vi "Clear Frame Filters.vi"(8 "error in":errorcluster, 11 "IMG_SRC in":refnum<class "IMG_SRC.lvclass">) -> (0 "error out":errorcluster, 3 "IMG_SRC out":refnum<class "IMG_SRC.lvclass">)   [LabVIEW 2018, in "IMG_SRC.lvlib" / "IMG_SRC.lvclass"]
uses:
  IMG_SRC.lvclass
  IMG_SRC.lvclass/IMG_SRC.ctl
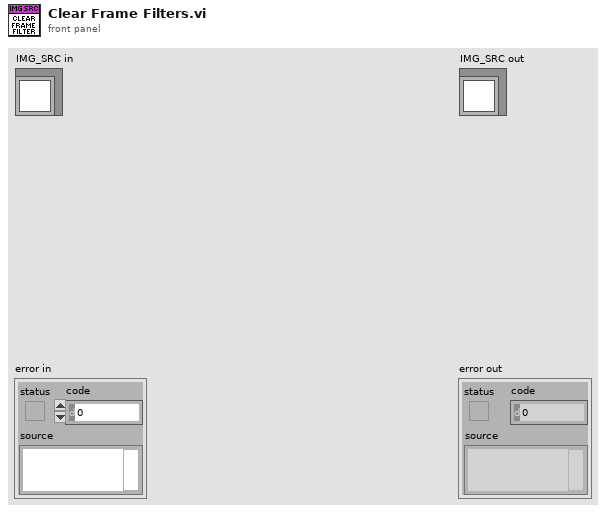
[diagram p1: front panel]
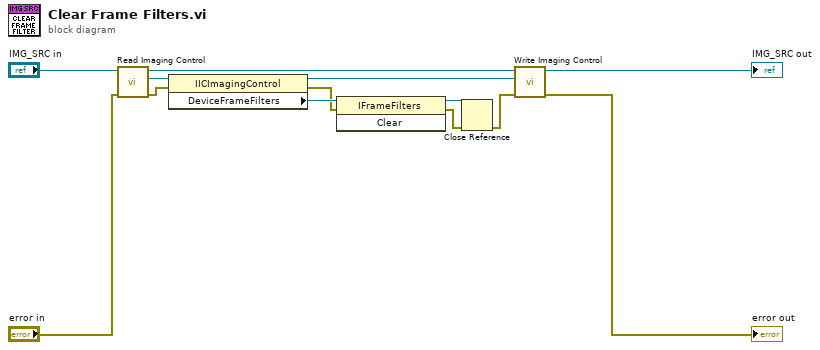
[diagram p0: block diagram]
diagram:
  n1 = call "Read Imaging Control.vi"("error in (no error)"="error in", "IMG_SRC in"="IMG_SRC in") -> ("error out"=w11:errorcluster, "Imaging Control"=w12:refnum<k7>, "IMG_SRC out"=w7:refnum<class "IMG_SRC.lvclass">)  [unwired: 7 in]
  n2 = property class="IICImagingControl"(reference=w12, error in=w11) -> (reference out=w8:refnum<k7>, error out=w9:errorcluster, "DeviceFrameFilters"=w10:refnum<k7>)
  n3 = invoke class="IFrameFilters" method="Clear"(reference=w10, error in=w9) -> (reference out=w3:refnum<k7>, error out=w2:errorcluster)  [unwired: 1 in, 1 out]
  n4 = Close Reference(reference=w3, error in (no error)=w2) -> (error out=w1:errorcluster)
  n5 = call "Write Imaging Control.vi"("error in (no error)"=w1, "Imaging Control"=w8, "IMG_SRC in"=w7) -> ("error out"=→"error out":errorcluster, "IMG_SRC out"=→"IMG_SRC out":refnum<class "IMG_SRC.lvclass">)  [unwired: 7 in]
